vi "WaitAnswer.vi"(4 "error in (no error)":errorcluster, 7 "VISA resource name in":refnum<visa-resource-name>) -> (0 "error out":errorcluster, 3 "VISA resource name out":refnum<visa-resource-name>)   [LabVIEW 2016]
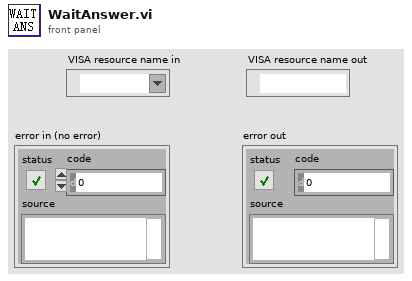
[diagram p1: front panel]
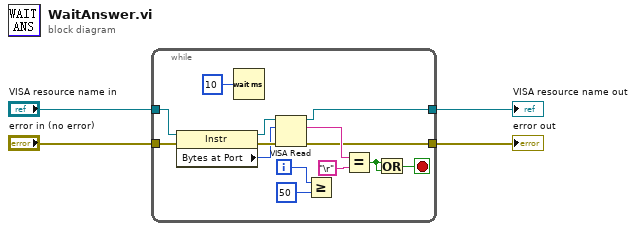
[diagram p0: block diagram]
diagram:
  n1 = while {
    tunnel: "VISA resource name in" -> [w13]
    tunnel: [w8] -> w3
    tunnel: [w6] -> w2
    tunnel: "error in (no error)" -> [w5]
    i -> [w17]
    stop <- w11 stop-if-true
    n2 = property class="Instr"(reference=w13, error in=w5) -> (reference out=w15:refnum<visa-resource-name>, error out=w14:errorcluster, "Bytes at Port"=w12:u32)
    n3 = Wait (ms)(milliseconds to wait=u32 10 ("等待时间（毫秒）")) -> ()  [unwired: 1 out]
    n4 = VISA Read(VISA resource name=w15, byte count=w12, error in (no error)=w14) -> (VISA resource name out=w8:refnum<visa-resource-name>, read buffer=w10:string, error out=w6:errorcluster)  [unwired: 1 out]
    n5 = Greater Or Equal?(x=w17, y=50) -> ()  [unwired: 1 out]
    n6 = Equal?(x=w10, y="\r") -> (x = y?=w7:bool)
    n7 = Or(x=w7, y=w7) -> (x .or. y?=w11:bool)
  }
  "VISA resource name out" <- w3
  "error out" <- w2
